vi "ADC Read Volts.vi"(8 "error in (no error)":errorcluster, 10 "ADC Channel Selection":T1, 11 "LINX-ADS1X15 in":refnum<class "LINX-ADS1X15.lvclass">) -> (0 "error out":errorcluster, 2 "ADC Volts":dbl, 3 "LINX-ADS1X15 out":refnum<class "LINX-ADS1X15.lvclass">)   [LabVIEW 2020, in "LINX-ADS1X15.lvclass"]
doc: "Reads the scaled ADC value in Volts from the ADS1X15 chip."
uses:
  LINX-ADS1X15.lvclass
  Channel Selection.ctl
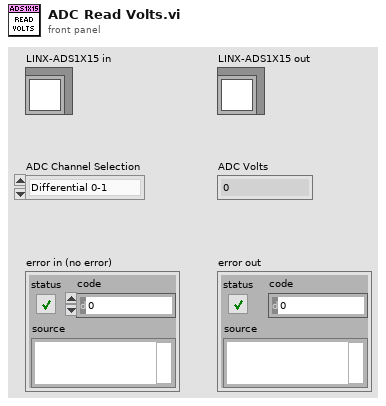
[diagram p1: front panel]
types:
  T1 = typedef "LINX-ADS1X15.lvclass/Channel Selection.ctl" = enum16{"Differential 0-1", "Differential 2-3", "Single Ended 0", "Single Ended 1", "Single Ended 2", "Single Ended 3"}
  T2 = typedef "LINX-ADS1X15.lvclass/Programmable Gain Selection.ctl" = enum16{"+/-6.144V (2/3)", "+/-4.096V (1)", "+/-2.048V (2)", "+/-1.024V (4)", "+/-0.512V (8)", "+/-0.256V (16)"}
  T3 = typedef "LINX-ADS1X15.lvclass/ADC Type Selection.ctl" = enum16{"ADS1015", "ADS1115"}
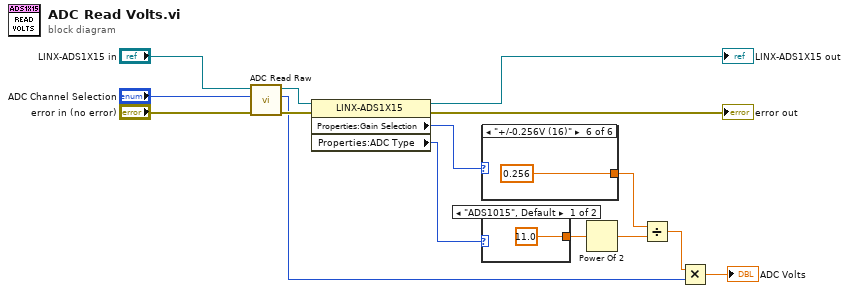
[diagram p0: block diagram]
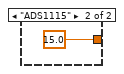
[diagram p2: hidden frame]
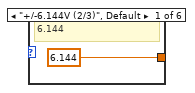
[diagram p3: hidden frame]
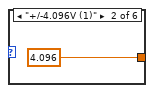
[diagram p4: hidden frame]
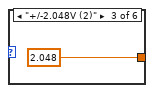
[diagram p5: hidden frame]
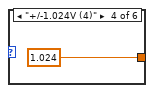
[diagram p6: hidden frame]
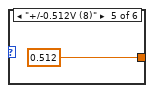
[diagram p7: hidden frame]
diagram:
  n1 = call-dynamic "ADC Read Raw.vi"("error in (no error)"="error in (no error)", "ADC Channel Selection"="ADC Channel Selection", "LINX-ADS1X15 in"="LINX-ADS1X15 in") -> ("error out"=w10:errorcluster, "ADC Raw"=w3:i16, "LINX-ADS1X15 out"=w15:refnum<class "LINX-ADS1X15.lvclass">)  [unwired: 6 in]
  n2 = property class="LINX-ADS1X15"(reference=w15, error in=w10) -> (reference out=→"LINX-ADS1X15 out":refnum<class "LINX-ADS1X15.lvclass">, error out=→"error out":errorcluster, "Properties:Gain Selection"=w8:T2, "Properties:ADC Type"=w1:T3)
  n3 = case shown="\"+/-0.256V (16)\"" w8 {
    tunnel: [6.144 4.096 2.048 1.024 0.512 0.256] -> w6
    frame "+/-6.144V (2/3)", Default {
      # "6.144"
    }
    frame "+/-4.096V (1)" {
    }
    frame "+/-2.048V (2)" {
    }
    frame "+/-1.024V (4)" {
    }
    frame "+/-0.512V (8)" {
    }
    frame "+/-0.256V (16)" {
    }
  }
  n4 = case shown="\"ADS1015\", Default" w1 {
    tunnel: [11.0 ("x") 15.0 ("x")] -> w7
    frame "ADS1015", Default {
    }
    frame "ADS1115" {
    }
  }
  n5 = Power Of 2(x=w7) -> (2^x=w5:dbl)
  n6 = Divide(x=w6, y=w5) -> (x/y=w4:dbl)
  n7 = Multiply(x=w4, y=w3) -> (x*y=→"ADC Volts":dbl)
